vi "BASE.GetConfig.vi"(8 "error in (no error)":errorcluster, 11 "BASE in":refnum<class "BASE.lvclass">) -> (0 "error out":errorcluster, 2 "Config":T1, 3 "BASE out":refnum<class "BASE.lvclass">)   [LabVIEW 2019, in "BASE.lvlib" / "BASE.lvclass"]
uses:
  BASE.lvclass
  config--cluster.ctl
  BASE.lvclass/BASE.ctl
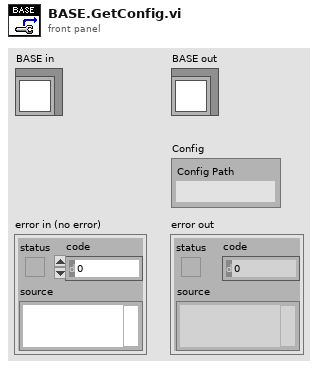
[diagram p1: front panel]
types:
  T1 = typedef "BASE.lvlib/BASE.lvclass/config--cluster.ctl" = cluster{"Config Path":path}
  T2 = typedef "BASE.lvlib/BASE.lvclass/privateData--reference.ctl" = refnum<data-value>
  T3 = typedef "BASE.lvlib/BASE.lvclass/privateData--cluster.ctl" = cluster{"config":T1, "Configured?":bool}
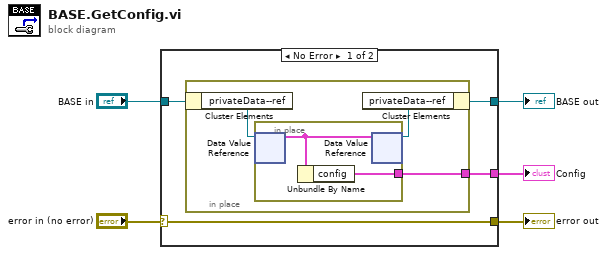
[diagram p0: block diagram]
diagram:
  n1 = case shown="No Error" "error in (no error)" {
    selector: "error in (no error)" -> [w9 w15]
    tunnel: [w9 w15] -> w4
    tunnel: [w6 w16] -> w1
    tunnel: "BASE in" -> [w7 w16]
    tunnel: [w8 _] -> w2
    frame No Error {
      n2 = in-place {
        in-place-border: [w12] -> w8
        n3 = in-place-cluster #1(w7) -> ("privateData--ref"=w11:T2)
        n4 = in-place {
          in-place-border: [w14] -> w12
          n5 = in-place-dvr #2(w11) -> (w13:T3)  [unwired: 1 out]
          n6 = Unbundle By Name(w13) -> ("config"=w14:T1)
          n7 = in-place-dvr #2(w13) -> (w10:T2)  [unwired: 1 out]
        }
        n8 = in-place-cluster #1("privateData--ref"=w10) -> (w6:refnum<class "BASE.lvclass">)
      }
    }
    frame Error {
    }
  }
  "error out" <- w4
  "BASE out" <- w1
  "Config" <- w2
